vi "libdaq_adc_extractChannelData.vi"(0 "error in (no error)":errorcluster, 2 "all_databuf":dbl[](array[numeric]), 3 "all_buflen":i32, 4 "ch_listlen":u8, 5 "ch_index":u8) -> (14 "error out":errorcluster, 18 "ch_databuf":dbl[](array[numeric]))   [LabVIEW 2022 SP3, in "libdaqVI.lvlib"]
uses:
  libdaqVI.lvlib
  dll/daqlib.dll
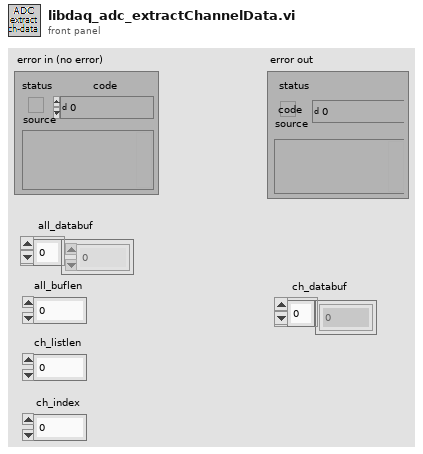
[diagram p1: front panel]
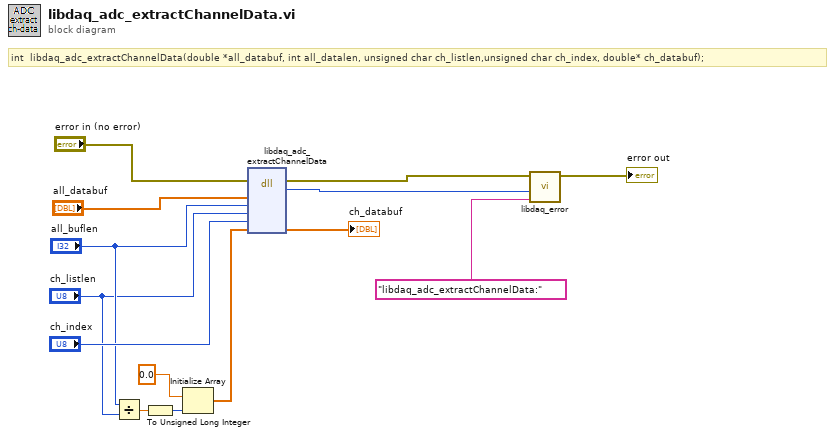
[diagram p0: block diagram]
diagram:
  # "int  libdaq_adc_extractChannelData(double *all_databuf, int all_datalen, unsigned char ch_listlen,unsigned char ch_index, double* ch_databuf);"
  n1 = Divide(x="all_buflen", y="ch_listlen") -> (x/y=w6:dbl)
  n2 = To Unsigned Long Integer(number=w6) -> (unsigned 32bit integer=w5:u32)
  n3 = Initialize Array(0.0, w5) -> (w10:dbl[])
  n4 = dll-call lib="D:/Labview_projects/DAQ_USB3212/libdaqVI/dll/daqlib.dll" fn="libdaq_adc_extractChannelData"(error in="error in (no error)", "all_databuf"="all_databuf", "all_buflen"="all_buflen", "ch_listlen"="ch_listlen", "ch_index"="ch_index", "ch_databuf"=w10) -> (error out=w2:errorcluster, "return type"=w3:i32, "ch_databuf"=→"ch_databuf":dbl[])  [unwired: 6 in, 1 out]
  n5 = call "libdaq_error.vi"("error source"="libdaq_adc_extractChannelData:" ("source"), "error code"=w3, "错误输入（无错误）"=w2) -> ("错误输出"=→"error out":errorcluster)  [unwired: 8 in]
